vi "VIQA Open File.vi"(8 "error in (no error)":errorcluster, 10 "Tag":string, 11 "Project in":refnum<vi>) -> (0 "error out":errorcluster)   [LabVIEW 2018, in "VI Quality.lvlib"]
doc: "This VI opens a file in its native application."
uses:
  VI Quality.lvlib
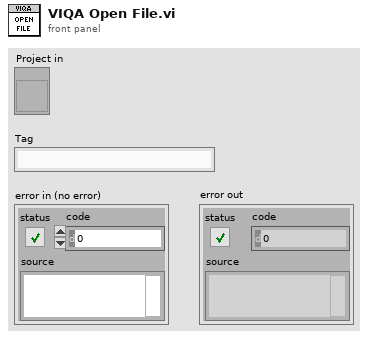
[diagram p1: front panel]
types:
  T1 = enum32{"invalid VI type", "Standard VI", "Control VI", "Global VI", "Polymorphic VI", "Configuration VI", "SubSystem", "Facade VI", "Method VI", "Statechart Diagram VI"}
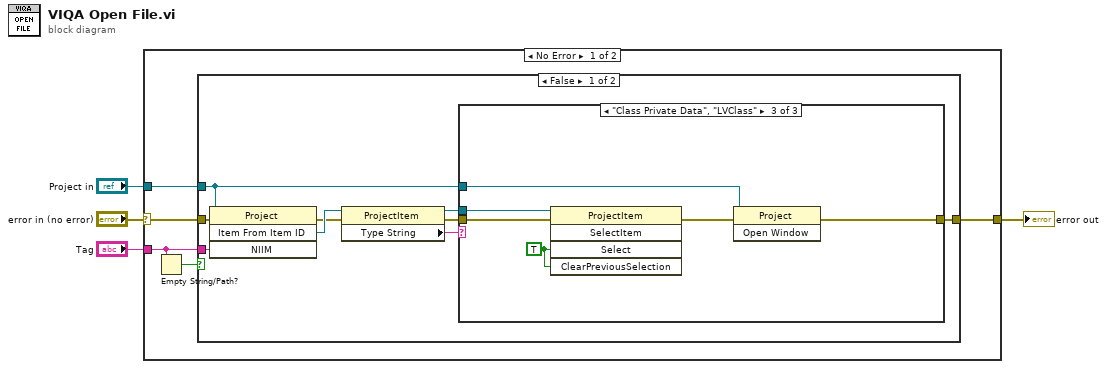
[diagram p0: block diagram]
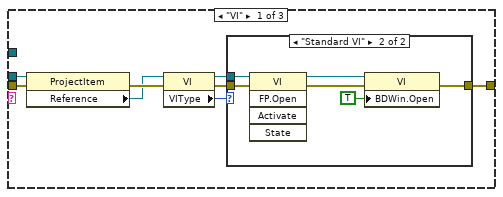
[diagram p2: hidden frame]
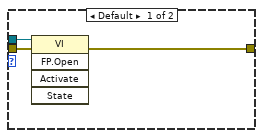
[diagram p3: hidden frame]
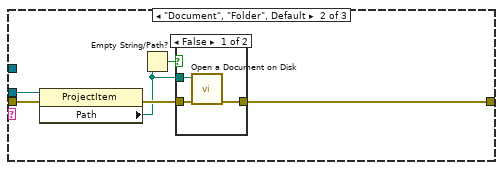
[diagram p4: hidden frame]
diagram:
  n1 = case shown="No Error" "error in (no error)" {
    selector: "error in (no error)" -> [w7 w53]
    tunnel: "Project in" -> [w9 _]
    tunnel: [w8 w53] -> w3
    tunnel: "Tag" -> [w6 _]
    frame No Error {
      n2 = Empty String/Path?(string/path=w6) -> (empty?=w5:bool)
      n3 = case shown="False" w5 {
        tunnel: w9 -> [w10 _]
        tunnel: [w16 w52] -> w8
        tunnel: w7 -> [w12 w52]
        tunnel: w6 -> [w11 _]
        frame False {
          n4 = invoke class="Project" method="Item From Item ID"(reference=w10, error in=w12, "NIIM"=w11) -> (error out=w13:errorcluster, "GetItemFromNIIM"=w14:refnum<vi>)  [unwired: 1 in, 2 out]
          n5 = property class="ProjectItem"(reference=w14, error in=w13) -> (reference out=w18:refnum<vi>, error out=w15:errorcluster, "Type String"=w17:string)
          n6 = case shown="\"Class Private Data\", \"LVClass\"" w17 {
            tunnel: w15 -> [w26 w40 w51]
            tunnel: [w23 w41 w47] -> w16
            tunnel: w18 -> [w25 w39 w50]
            tunnel: w10 -> [_ _ w46]
            frame "VI" {
              n7 = property class="ProjectItem"(reference=w25, error in=w26) -> (error out=w24:errorcluster, "Reference"=w21:refnum<vi>)  [unwired: 1 out]
              n8 = property class="VI"(reference=w21, error in=w24) -> (reference out=w20:refnum<vi>, error out=w22:errorcluster, "VIType"=w19:T1)
              n9 = case shown="\"Standard VI\"" w19 {
                tunnel: [w29 w32] -> w23
                tunnel: w22 -> [w28 w34]
                tunnel: w20 -> [w27 w33]
                frame Default {
                  n10 = invoke class="VI" method="FP.Open"(reference=w27, error in=w28) -> (error out=w29:errorcluster)  [unwired: 3 in, 4 out]
                }
                frame "Standard VI" {
                  n11 = invoke class="VI" method="FP.Open"(reference=w33, error in=w34) -> (reference out=w31:refnum<vi>, error out=w35:errorcluster)  [unwired: 3 in, 3 out]
                  n12 = property class="VI"(reference=w31, error in=w35, "BDWin.Open"=TRUE ("Block Diagram Window:Open")) -> (error out=w32:errorcluster)  [unwired: 1 out]
                }
              }
            }
            frame "Document", "Folder", Default {
              n13 = property class="ProjectItem"(reference=w39, error in=w40) -> (error out=w38:errorcluster, "Path"=w37:path)  [unwired: 1 out]
              n14 = Empty String/Path?(string/path=w37) -> (empty?=w36:bool)
              n15 = case shown="False" w36 {
                tunnel: [w44 w45] -> w41
                tunnel: w38 -> [w43 w45]
                tunnel: w37 -> [w42 _]
                frame False {
                  n16 = call <vilib>:"Open a Document on Disk.vi"("error in (no error)"=w43, "document path"=w42) -> ("error out"=w44:errorcluster)  [unwired: 5 in]
                }
                frame True {
                }
              }
            }
            frame "Class Private Data", "LVClass" {
              w49 = TRUE ("Select")
              n17 = invoke class="ProjectItem" method="SelectItem"(reference=w50, error in=w51, "Select"=w49, "ClearPreviousSelection"=w49) -> (error out=w48:errorcluster)  [unwired: 1 in, 4 out]
              n18 = invoke class="Project" method="Open Window"(reference=w46, error in=w48) -> (error out=w47:errorcluster)  [unwired: 1 in, 2 out]
            }
          }
        }
        frame True {
        }
      }
    }
    frame Error {
    }
  }
  "error out" <- w3
